vi "ParsedivClick.vi"(0 "Text in":string, 1 "HTML in":string) -> (2 "Text out":string, 3 "Color":u32(colorbox), 4 "success?":bool, 5 "HTML out":string)   [LabVIEW 2016]
doc: "Parses div and color codes"
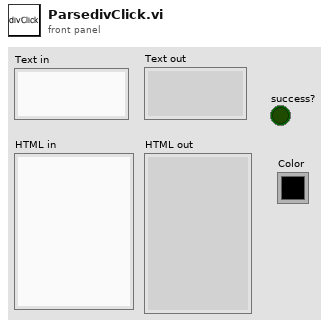
[diagram p1: front panel]
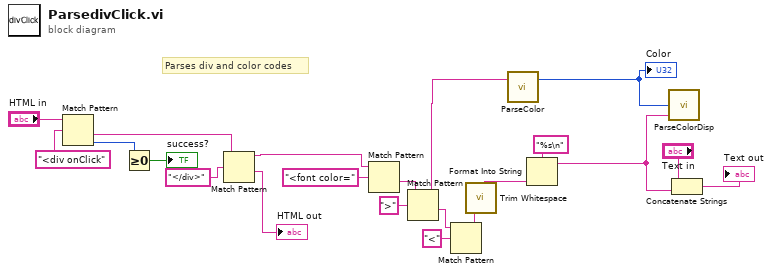
[diagram p0: block diagram]
diagram:
  # "Parses div and color codes"
  n1 = Match Pattern(string="HTML in", regular expression="<div onClick") -> (after substring=w19:string, offset past match=w7:i32)  [unwired: 1 in, 2 out]
  n2 = Greater Or Equal To 0?(x=w7) -> (x >= 0?=→"success?":bool)
  n3 = Match Pattern(string=w19, regular expression="</div>") -> (before substring=w21:string, after substring=→"HTML out":string)  [unwired: 1 in, 2 out]
  n4 = Match Pattern(string=w21, regular expression="<font color=") -> (after substring=w12:string)  [unwired: 1 in, 3 out]
  n5 = Match Pattern(string=w12, regular expression=">") -> (before substring=w5:string, after substring=w14:string)  [unwired: 1 in, 2 out]
  n6 = Match Pattern(string=w14, regular expression="<") -> (before substring=w16:string)  [unwired: 1 in, 3 out]
  n7 = call <vilib>:"Trim Whitespace.vi"("string"=w16) -> ("trimmed string"=w17:string)  [unwired: 1 in]
  n8 = call "ParseColor.vi"("HTML in"=w5) -> ("Color"=w4:u32)  [unwired: 2 in]
  "Color" <- w4
  n9 = Format Into String(format string="%s\n" ("regular expression"), w17) -> (resulting string=w3:string)  [unwired: 2 in, 1 out]
  n10 = call "ParseColorDisp.vi"("text"=w3, "text color(black)"=w4) -> ()  [unwired: 2 in, 1 out]
  n11 = Concatenate Strings("Text in", w3) -> (→"Text out":string)
